vi "get all VIs in SciScan directory.vi"(11 "keep GFG unlocked":bool) -> (3 "All Files in Dir":path[](array[path]))   [LabVIEW 2012]
panel:
  out "size(s)":i32
  out "error out":errorcluster
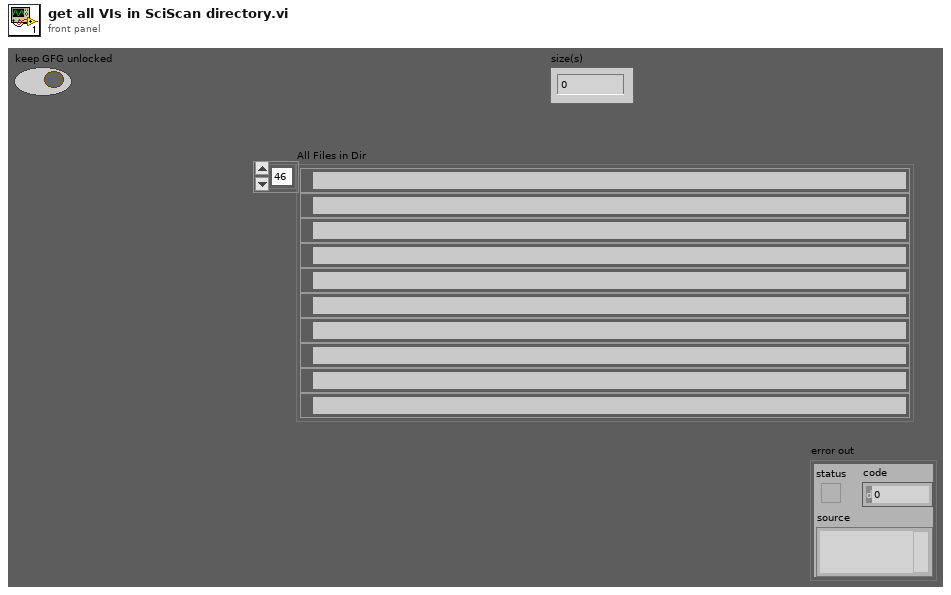
[diagram p1: front panel]
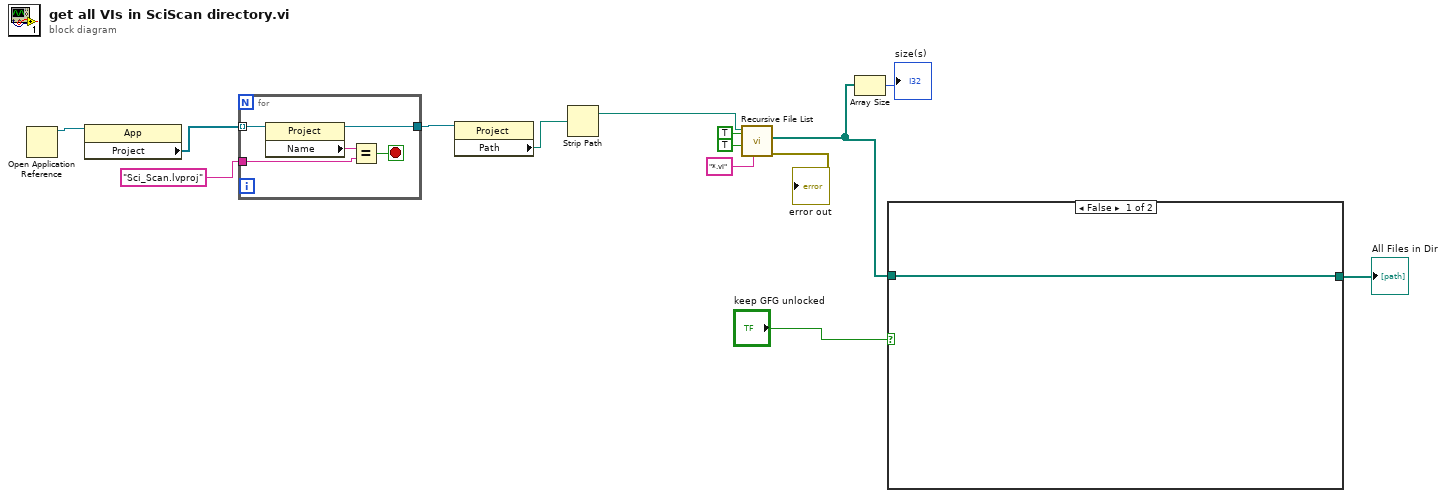
[diagram p0: block diagram]
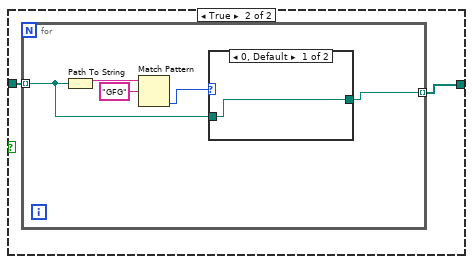
[diagram p2: hidden frame]
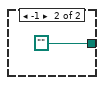
[diagram p3: hidden frame]
diagram:
  n1 = Open Application Reference() -> (3:w14:refnum<vi>)  [unwired: 4 in, 1 out]
  n2 = property class="App"(reference=w14) -> ("Project"=w13:refnum<vi>[])  [unwired: 1 in, 2 out]
  n3 = for {
    tunnel: w13 -> [w19] mode=indexing
    tunnel: "Sci_Scan.lvproj" ("Name") -> [w17]
    tunnel: [w15] -> w11
    stop <- w16 stop-if-true
    n4 = property class="Project"(reference=w19) -> (reference out=w15:refnum<vi>, "Name"=w18:string)  [unwired: 1 in, 1 out]
    n5 = Equal?(x=w18, y=w17) -> (x = y?=w16:bool)
  }
  n6 = property class="Project"(reference=w11) -> ("Path"=w8:path)  [unwired: 1 in, 2 out]
  n7 = Strip Path(path=w8) -> (stripped path=w6:path)  [unwired: 1 out]
  n8 = call <vilib>:"Recursive File List.vi"("pattern"="*.vi", "Continue Recursing on Error? (F)"=TRUE, "Treat LLBs as Folders?"=TRUE, "Folder Path"=w6) -> ("error out"=→"error out":errorcluster, "All Files in Dir"=w3:path[])  [unwired: 3 in, 3 out]
  n9 = Array Size(array=w3) -> (size(s)=→"size(s)":i32)
  n10 = case shown="False" "keep GFG unlocked" {
    tunnel: w3 -> [w20 w22]
    tunnel: [w20 w21] -> w2
    frame False {
    }
    frame True {
      n11 = for {
        tunnel: w22 -> [w23] mode=indexing
        tunnel: [w24] -> w21 mode=indexing
        n12 = Path To String(path=w23) -> (string=w27:string)
        n13 = Match Pattern(string=w27, regular expression="GFG") -> (offset past match=w25:i32)  [unwired: 1 in, 3 out]
        n14 = case shown="0, Default" w25 {
          tunnel: [w28 path ""] -> w24
          tunnel: w23 -> [w28 _]
          frame 0, Default {
          }
          frame -1 {
          }
        }
      }
    }
  }
  "All Files in Dir" <- w2
